vi "Check Is Middle Reached.vi"(10 "Middle y":sgl, 11 "Current Row":i32) -> (3 "Reached Middle":bool)   [LabVIEW 2020, in "Raster (FPGA).lvlib"]
uses:
  Raster (FPGA).lvlib
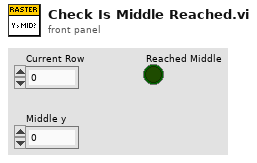
[diagram p1: front panel]
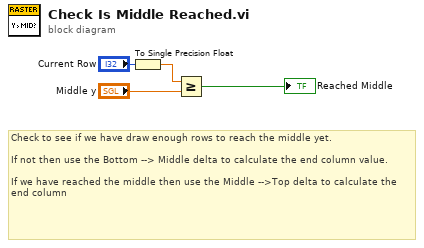
[diagram p0: block diagram]
diagram:
  # "Check to see if we have draw enough rows to reach the middle yet.\n\nIf not then use the Bottom --> Middle delta to calculate the end column value.\n\nIf we have reached the middle then use the Middle -->Top delta to calculate the end column"
  n1 = To Single Precision Float(number="Current Row") -> (single precision float=w1:sgl)
  n2 = Greater Or Equal?(x=w1, y="Middle y") -> (x >= y?=→"Reached Middle":bool)
